vi "DAQ_Launcher.vi"(6 "ShowPanel":bool, 8 "error in (no error)":errorcluster, 9 "Debug":bool, 10 "Context":refnum<vi>, 11 "ModuleName":string) -> (0 "error out":errorcluster, 3 "Message Enqueuer out":refnum<class "Message Enqueuer.lvclass">)   [LabVIEW 2025, in "DAQ_API.lvlib"]
uses:
  DAQ_API.lvlib
  DAQ_Module/DAQ_Module/DAQ_Module/DAQ_Module.lvclass
  <vilib>/ActorFramework/Actor/Actor.lvclass
  Msg.ctl
  85d80bde-40ef-48e3-8d40-cfa78b1247cc.vi
  Module/Module/Module Messages/CoreComm Msg/CoreComm Msg.lvclass
  <vilib>/ActorFramework/Message Enqueuer/Message Enqueuer.lvclass
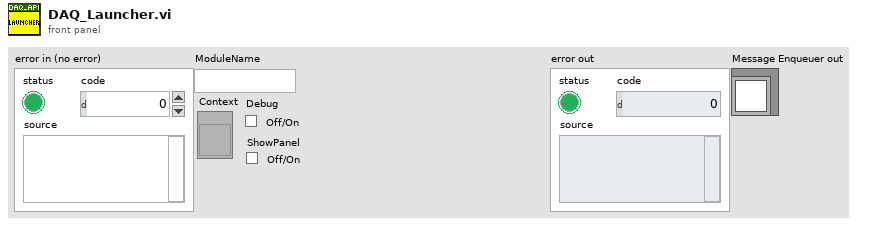
[diagram p1: front panel]
types:
  T1 = typedef "Msg.ctl" = string
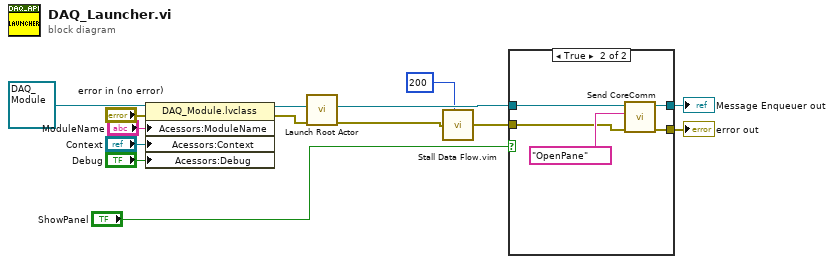
[diagram p0: block diagram]
diagram:
  n1 = property class="DAQ_Module.lvclass"(reference=refnum<class "DAQ_Module.lvclass"> refnum ("DAQ_Module.lvlib:DAQ_Module.lvclass"), error in="error in (no error)", "Acessors:ModuleName"="ModuleName", "Acessors:Context"="Context", "Acessors:Debug"="Debug") -> (reference out=w9:refnum<class "DAQ_Module.lvclass">, error out=w3:errorcluster)
  n2 = call <vilib>:"Launch Root Actor.vi"("error in (no error)"=w3, "Actor"=w9) -> ("error out"=w7:errorcluster, "Actor's Enqueuer"=w8:refnum<class "Message Enqueuer.lvclass">)  [unwired: 8 in]
  n3 = call "Stall Data Flow.vim"("value in"=w7, "milliseconds to wait"=u32 200) -> ("value out"=w6:errorcluster)  [unwired: 1 out]
  n4 = case shown="True" "ShowPanel" {
    tunnel: w8 -> [w15 w19]
    tunnel: w6 -> [w16 w17]
    tunnel: [w16 w20] -> w2
    tunnel: [w15 w21] -> w1
    frame False {
    }
    frame True {
      n5 = call "Send CoreComm.vi"("error in (no error)"=w17, "Msg"=T1 "OpenPane", "Message Enqueuer"=w19) -> ("error out"=w20:errorcluster, "Message Enqueuer out"=w21:refnum<class "Message Enqueuer.lvclass">)  [unwired: 7 in]
    }
  }
  "error out" <- w2
  "Message Enqueuer out" <- w1
